vi "to_string.vi"(7 "Serialized by PLC? (F)":bool, 8 "error_in":errorcluster, 9 "string_length":i32, 10 "variable_start_index":i32, 11 "byte_array":u8[](array[numeric])) -> (0 "error_out":errorcluster, 3 "string":string)   [LabVIEW 2020]
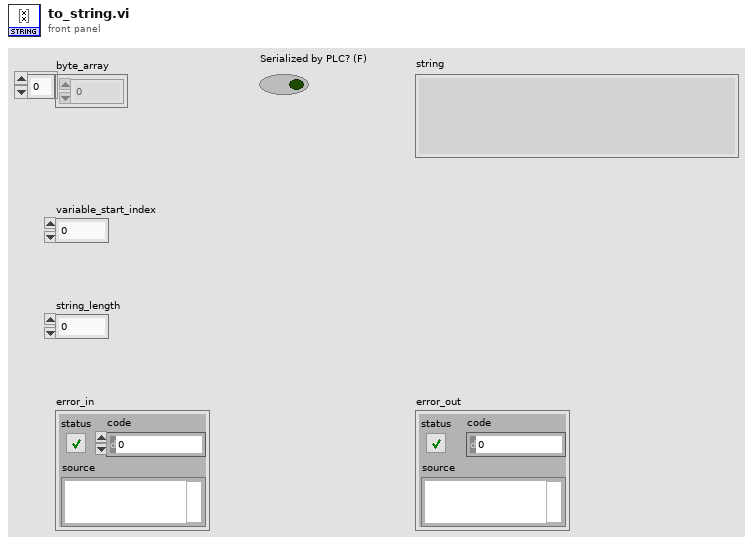
[diagram p1: front panel]
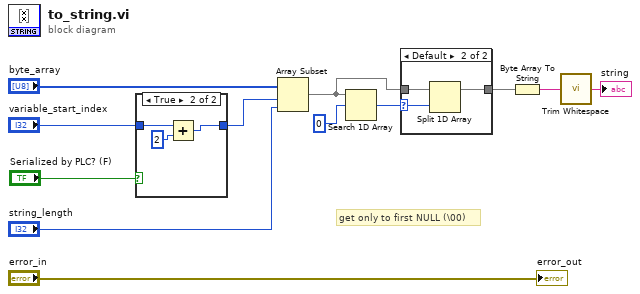
[diagram p0: block diagram]
diagram:
  # "get only to first NULL (\\00)"
  n1 = case shown="True" "Serialized by PLC? (F)" {
    tunnel: "variable_start_index" -> [w13 w16]
    tunnel: [w13 w15] -> w1
    frame False {
    }
    frame True {
      n2 = Add(x=w16, y=2) -> (x+y=w15:i32)
    }
  }
  n3 = Array Subset(array="byte_array", index=w1, length="string_length") -> (w5:u8[])
  n4 = Search 1D Array(1D array=w5, element=u8 0) -> (index of element=w6:i32)  [unwired: 1 in]
  n5 = case shown="Default" w6 {
    selector: w6 -> [_ w20]
    tunnel: w5 -> [w17 w19]
    tunnel: [w17 w18] -> w4
    frame -1 {
    }
    frame Default {
      n6 = Split 1D Array(array=w19, index=w20) -> (first subarray=w18:u8[])  [unwired: 1 out]
    }
  }
  n7 = Byte Array To String(unsigned byte array=w4) -> (string=w9:string)
  n8 = call <vilib>:"Trim Whitespace.vi"("string"=w9) -> ("trimmed string"=→"string":string)  [unwired: 1 in]
  "error_out" <- "error_in"
